vi "FFT(FPGA).vi"() -> ()   [LabVIEW 2019]
uses:
  <vilib>/rvi/Analysis/measure/FFT/simModelSupport/niFPGA FFT Outside SCTL Sim Properties.ctl
  <vilib>/rvi/Analysis/measure/FFT/simModelSupport/niFPGA FFT Sim Types.ctl
  <vilib>/rvi/Analysis/measure/FFT/simModelSupport/niFpgaFFTSimArithmeticProperties.ctl
  <vilib>/rvi/Analysis/measure/FFT/simModelSupport/niFpgaFFTSimDfxp.ctl
  <vilib>/fxp/LVFixedPointQuantizationPolicyTypeDef.ctl
  <vilib>/rvi/Emulation/niFpgaGetClockAttributes.vi
  <vilib>/rvi/Emulation/niFpgaSctlEmulationGetInTimedLoop.vi
  <vilib>/rvi/Emulation/niFpgaEmulationReportErrorSimple.vi
  <vilib>/rvi/eio/common/nirviEmuTemplateMethod_errors.vi
  <vilib>/rvi/Emulation/niFpgaEmulationIsFPGAContextNoSignature.vi
  <vilib>/rvi/DataTransferAndStorage/Container/Common/niFpgaContainerGetUniqueNameForEmu.vi
  <vilib>/rvi/Memory/Memory_Emulation/niFpgaMemoryEmulationCacheClearOnFirstRun.vi
  <vilib>/rvi/Memory/Memory_Emulation/nirvimemoryEmulationManagerCache_MakeExclusive.vi
  <vilib>/rvi/Memory/Memory_Emulation/niFpgaMemoryEmulationValidateCache.vi
  <vilib>/rvi/Memory/Memory_Emulation/nirvimemoryEmulationManagerCache_InsertValue.vi
  <vilib>/Utility/error.llb/Clear Errors.vi
  <vilib>/rvi/Memory/Memory_Emulation/nirvimemoryEmulationManagerCache_ReleaseExclusive.vi
  <vilib>/rvi/Memory/Memory_Emulation/nirvimemoryEmulationManagerCache_GetValue.vi
  <vilib>/rvi/Memory/Memory_Emulation/nirvimemoryEmulationManagerCache_SetValue.vi
  <vilib>/rvi/Emulation/niFpgaProcessEmulError.vi
  <vilib>/rvi/Emulation/niFpgaCriticalErrorInLSC.vi
  <vilib>/rvi/Analysis/measure/FFT/simModelSupport/niFpgaFFTSimModelOutsideSCTLCore.vi
  <vilib>/rvi/interface/RandomDataEmulation/niFpgaRandomDataHandleErrors.vi
  <vilib>/eio/EIONode/EIONode.xnode
  <vilib>/rvi/DataTransferAndStorage/Container/XNode/niFpgaContainer.xnode
  <vilib>/rvi/DataTransferAndStorage/Register/Emulation/niFpgaRegisterEmulation.vi
  <vilib>/rvi/Analysis/measure/FFT/XNode/niFpgaFFT.xnode
  <vilib>/rvi/interface/RandomDataEmulation/nirviRandomDataFpgaReadWriteTemplate.vi
panel:
  in  "LED3":bool
  in  "LED2":bool
  in  "LED1":bool
  in  "LED0":bool
  in  "stop":bool
  in  "Initialize":bool
  in  "Sine wave properties":T1={"Frequency (periods/tick)"=0.0002500000409781933, "Phase offset (periods)"=0.0, "Scale factor"=1.0, "Amplitude offset"=0.0}
  in  "Count(mSec)":u32
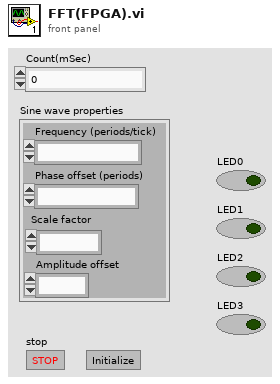
[diagram p1: front panel]
types:
  T1 = cluster{"Frequency (periods/tick)":fxp<+,32,0>, "Phase offset (periods)":fxp<+,32,0>, "Scale factor":fxp<+,12,1>, "Amplitude offset":fxp<+/-,16,12>}
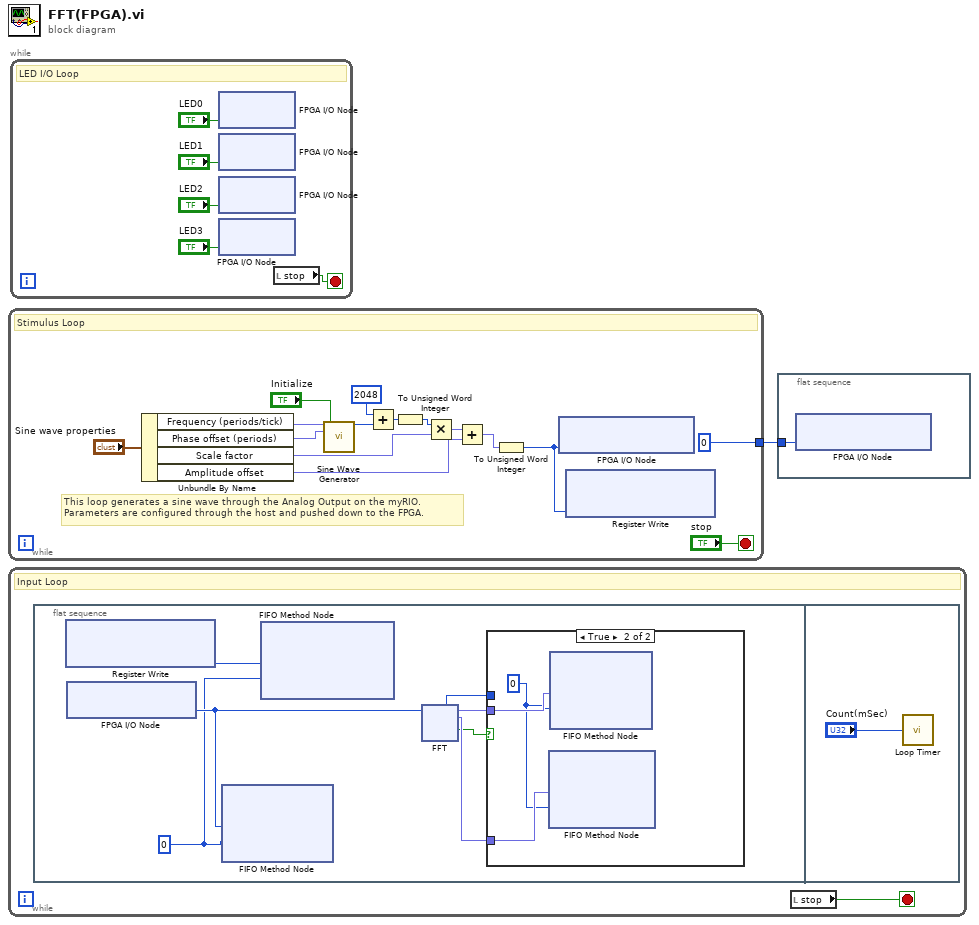
[diagram p0: block diagram]
diagram:
  n1 = while {
    tunnel: [i16 0 ("ConnectorC/AO0")] -> w1
    stop <- "stop" stop-if-true
    # "This loop generates a sine wave through the Analog Output on the myRIO.\nParameters are configured through the host and pushed down to the FPGA."
    # "Stimulus Loop"
    n2 = Unbundle By Name("Sine wave properties") -> ("Frequency (periods/tick)"=w12:fxp<+,32,0>, "Phase offset (periods)"=w11:fxp<+,32,0>, "Scale factor"=w14:fxp<+,12,1>, "Amplitude offset"=w13:fxp<+/-,16,12>)
    n3 = call "Sine Wave Generator"("frequency (periods/tick)"=w12, "reset"="Initialize", "phase offset (periods)"=w11) -> ("sine out"=w8:i16)  [unwired: 12 in]
    n4 = Add(x=i16 2048, y=w8) -> (x+y=w6:i16)
    n5 = To Unsigned Word Integer(number=w6) -> (unsigned 16bit integer=w5:u16)
    n6 = Multiply(x=w5, y=w14) -> (x*y=w10:fxp<+,28,17>)
    n7 = Add(x=w10, y=w13) -> (x+y=w4:fxp<+,12,12>)
    n8 = To Unsigned Word Integer(number=w4) -> (unsigned 16bit integer=w2:u16)
    n9 = xnode "FPGA I/O Node"("ConnectorC/AO0"=w2) -> ()  [unwired: 1 in, 1 out]
    n10 = xnode "Register Write"("Data"=w2) -> ()  [unwired: 1 in, 1 out]
  }
  n11 = while {
    stop <- w17 stop-if-true
    # "Input Loop"
    n12 = flat-sequence {
      frame #0 {
        w19 = 0 ("Timeout")
        n13 = xnode "Register Write"() -> ("Data"=w18:i16)  [unwired: 1 in, 1 out]
        n14 = xnode "FPGA I/O Node"() -> ("ConnectorC/AI0"=w20:i16)  [unwired: 1 in, 1 out]
        n15 = xnode ("FIFO Method Node")("Element"=w20, "Timeout"=w19) -> ()  [unwired: 1 in, 2 out]
        n16 = xnode ("FIFO Method Node")("Element"=w18, "Timeout"=w19) -> ()  [unwired: 1 in, 2 out]
        n17 = xnode "FFT"("real data in"=w20) -> ("data index"=w23:u16, "real data out"=w24:fxp<+/-,27,27>, "imaginary data out"=w22:fxp<+/-,27,27>, "output valid"=w21:bool)  [unwired: 2 in]
        n18 = case shown="True" w21 {
          tunnel: w24 -> [_ w27]
          tunnel: w23 -> [_ _]
          tunnel: w22 -> [_ w26]
          frame False {
          }
          frame True {
            w25 = 0 ("Timeout")
            n19 = xnode ("FIFO Method Node")("Element"=w26, "Timeout"=w25) -> ()  [unwired: 1 in, 2 out]
            n20 = xnode ("FIFO Method Node")("Element"=w27, "Timeout"=w25) -> ()  [unwired: 1 in, 2 out]
          }
        }
      }
      frame #1 {
        n21 = call "Loop Timer"("Count(uSec)"="Count(mSec)") -> ()  [unwired: 1 out]
      }
    }
    n22 = local read "stop"() -> (w17:bool)
  }
  n23 = while {
    stop <- w53 stop-if-true
    # "LED I/O Loop"
    n24 = xnode "FPGA I/O Node"("LED0"="LED0") -> ()  [unwired: 1 in, 1 out]
    n25 = xnode "FPGA I/O Node"("LED1"="LED1") -> ()  [unwired: 1 in, 1 out]
    n26 = xnode "FPGA I/O Node"("LED2"="LED2") -> ()  [unwired: 1 in, 1 out]
    n27 = xnode "FPGA I/O Node"("LED3"="LED3") -> ()  [unwired: 1 in, 1 out]
    n28 = local read "stop"() -> (w53:bool)
  }
  n29 = flat-sequence {
    tunnel: w1 -> [w54]
    frame #0 {
      n30 = xnode "FPGA I/O Node"("ConnectorC/AO0"=w54) -> ()  [unwired: 1 in, 1 out]
    }
  }
